vi "Unpack Subscription Request.vi"(11 "SubscriptionRequest in":refnum<class "SubscriptionRequest.lvclass">) -> (0 "Subscription Policy":T1, 1 "Unique Subscriber ID":string, 2 "Type":variant, 3 "Datum Name":string)   [LabVIEW 2015, in "IMediator.lvlib" / "SubscriptionRequest.lvclass"]
doc: "<License>\nCopyright © 2017 Composed Systems, LLC | All rights reserved\nwww.composed.io\n\nAuthor: Ethan Stern <ethan.stern@composed.io>\n\nThis software is provided \"AS IS\" WITHOUT WARRANTIES, either express or implied, AND IS FOR EDUCATIONAL PURPOSES ONLY.\n</License>"
uses:
  SubscriptionRequest.lvclass
  ISubscriptionPolicy/ISubscriptionPolicy Reference.ctl
  ISubscriptionPolicy/ISubscriptionPolicy.lvclass
  SubscriptionRequest.lvclass/SubscriptionRequest.ctl
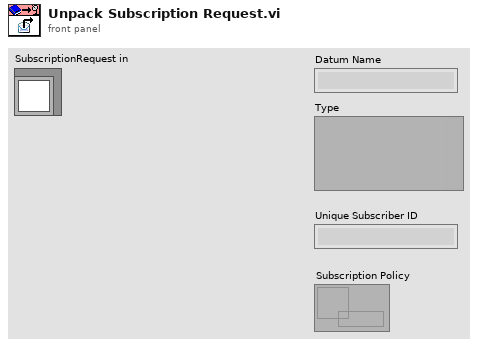
[diagram p1: front panel]
types:
  T1 = typedef "IMediator.lvlib/ISubscriptionPolicy.lvclass/ISubscriptionPolicy Reference.ctl" = refnum<data-value>
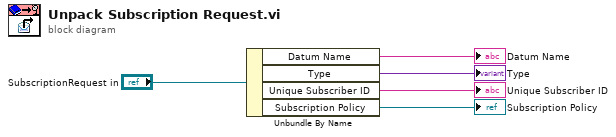
[diagram p0: block diagram]
diagram:
  n1 = Unbundle By Name("SubscriptionRequest in") -> ("Datum Name"=→"Datum Name":string, "Type"=→"Type":variant, "Unique Subscriber ID"=→"Unique Subscriber ID":string, "Subscription Policy"=→"Subscription Policy":T1)
